vi "multi-mode-acquisition.vi"() -> ()   [LabVIEW 2014]
uses:
  camera test/SubVIs/Initilize Globals.vi
  <vilib>/vision/Image Controls.llb/IMAQ Image.ctl
  Glimpse-master/Glimpse core/Seq file v 1/Offset.ctl
  Glimpse-master/Glimpse core/Seq file v 1/file number.ctl
  Glimpse-master/Glimpse core/Seq file v 1/Offset table.ctl
  camera test/SubVIs/ctt's/Video acquisition state1.ctl
  Shutter Control/Shutter SubVis/Global Shutter Variables - SubVI.vi
  Shutter Control/Shutter SubVis/user event shutter global.ctl
  Shutter Control/Shutter SubVis/laser shutters.ctl
panel:
  in  "Max. number of acquisition files":i8(slide)=10 scale=0.0..50.0
  in  "Acquisition Protocol":T2(array[cluster])
  in  "Quit":bool
  in  "Start":bool
  in  "Acquisition Parameters":T3={"Readout Mode"=enum."Image", "Set Acquisition Mode"=enum."Single Scan", "Trigger Mode"=enum."Internal", "Exposure Time (s)"=1.0, "Accumulation Cycle (s)"=0.0, "Kinetic Cycle Time (s)"=1.0, "Number of Kinetics"=1, "Number of Accumulations"=1, "Set VS Speed"=1, "Pixel Rate"=enum."Standard CCD 3 Mhz 14 bits", "V Shift Amplitude"=enum."+1", "Preamp Gain"=enum."1.0"}
  in  "Image Size":T4={"H Bin"=1.0, "V Bin"=1.0, "Left"=1.0, "Right"=1024.0, "Top"=1.0, "Bottom"=1024.0} {"V Bin" min=0.0; "H Bin" min=0.0 step=1.0}
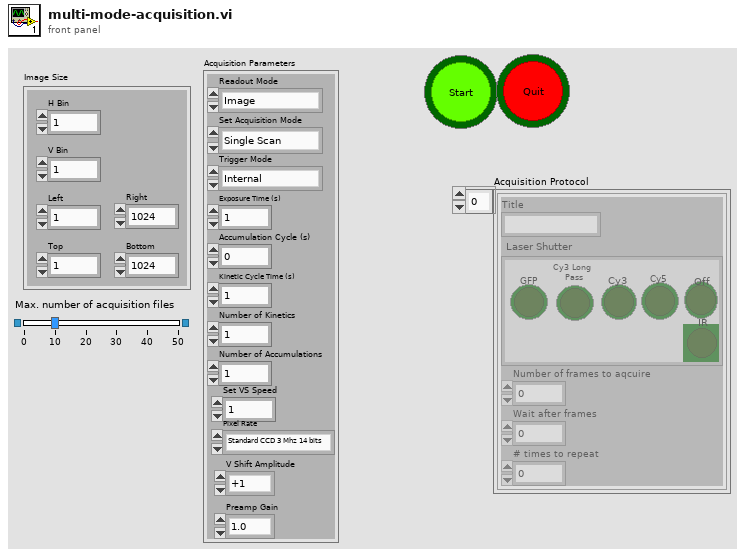
[diagram p1: front panel]
types:
  T1 = typedef "laser shutters.ctl" = enum32{"No Selection", "GFP", "Cy3 Long \nPass", "Cy3", "Cy5", "Off", "IR"}
  T2 = cluster{"Title":string, "Laser Shutter":T1, "Number of frames to aqcuire":dbl, "Wait after frames":dbl, "# times to repeat":dbl}[]
  T3 = cluster{"Readout Mode":enum16{"Full Vertical Binning", "Multi-Track", "Random-Track", "Single-Track", "Image"}, "Set Acquisition Mode":enum16{"(do nothing)", "Single Scan", "Accumulate", "Kinetics", "Fast Kinetics", "Run till abort"}, "Trigger Mode":enum16{"Internal", "External"}, "Exposure Time (s)":dbl, "Accumulation Cycle (s)":dbl, "Kinetic Cycle Time (s)":dbl, "Number of Kinetics":i32, "Number of Accumulations":i32, "Set VS Speed":i32, "Pixel Rate":enum16{"EM CCD 10 Mhz 14 bits", "EM CCD 5 Mhz 14 bits", "EM CCD 3 Mhz 14 bits", "EM CCD 1 Mhz 16 bits", "Standard CCD 3 Mhz 14 bits", "Standard CCD 1 Mhz 16 bits"}, "V Shift Amplitude":enum16{"normal", "+1", "+2", "+3", "+4"}, "Preamp Gain":enum16{"1.0", "2.4", "5.0"}}
  T4 = cluster{"H Bin":dbl, "V Bin":dbl, "Left":dbl, "Right":dbl, "Top":dbl, "Bottom":dbl}
  T5 = typedef "Video acquisition state1.ctl" = cluster{"Pixel depth":enum32{"8 bits", "16 bits", "Float", "Complex", "RGB Chunky", "Compressed"}, "Width":dbl, "Height":dbl, "Buffer":T6, "Frames Acquired":u32, "Time of 1st frame":dbl, "TTB element zero":u32, "File Offsets Array":T7, "TTB Array":u32[], "Sum Image (for averaging)":T6, "Time at end of last acquisition (ms)":u32, "Filter array":u16[], "Flow rate array":dbl[], "Temperature array":dbl[], "Field array":u16[], "Lasers array":u16[][], "Stage xyz array":dbl[][]}
  T6 = typedef "IMAQ Image.ctl" = refnum<image>
  T7 = typedef "Offset table.ctl" = cluster{"offset":T8, "file number":T9}[]
  T8 = typedef "Offset.ctl" = i32
  T9 = typedef "file number.ctl" = u8
  T10 = typedef "user event shutter global.ctl" = cluster{"Camera Shutter":bool, "Wheel Speed":u8, "Laser Shutter":enum32{"No Selection", "GFP", "Cy3 Long \nPass", "Cy3", "Cy5", "Off", "IR"}}
  T11 = cluster{"Frame Size (bytes)":i32, "Max Time (min)":i32, "Max Frames":i32, "Frames per acquisition file":i32, "Max time (s)":i32, "Max Space Req'd. (Gb)":dbl}
  T12 = typedef "acquisition control.ctl" = cluster{"H Bin":dbl, "V Bin":dbl, "Left":dbl, "Right":dbl, "Top":dbl, "Bottom":dbl}
  T13 = cluster{"Sequence files directory path":path, "Sequence files refnum array":refnum<file>[]}
  T14 = enum32{"No Selection", "GFP", "Cy3 Long \nPass", "Cy3", "Cy5", "Off", "IR"}
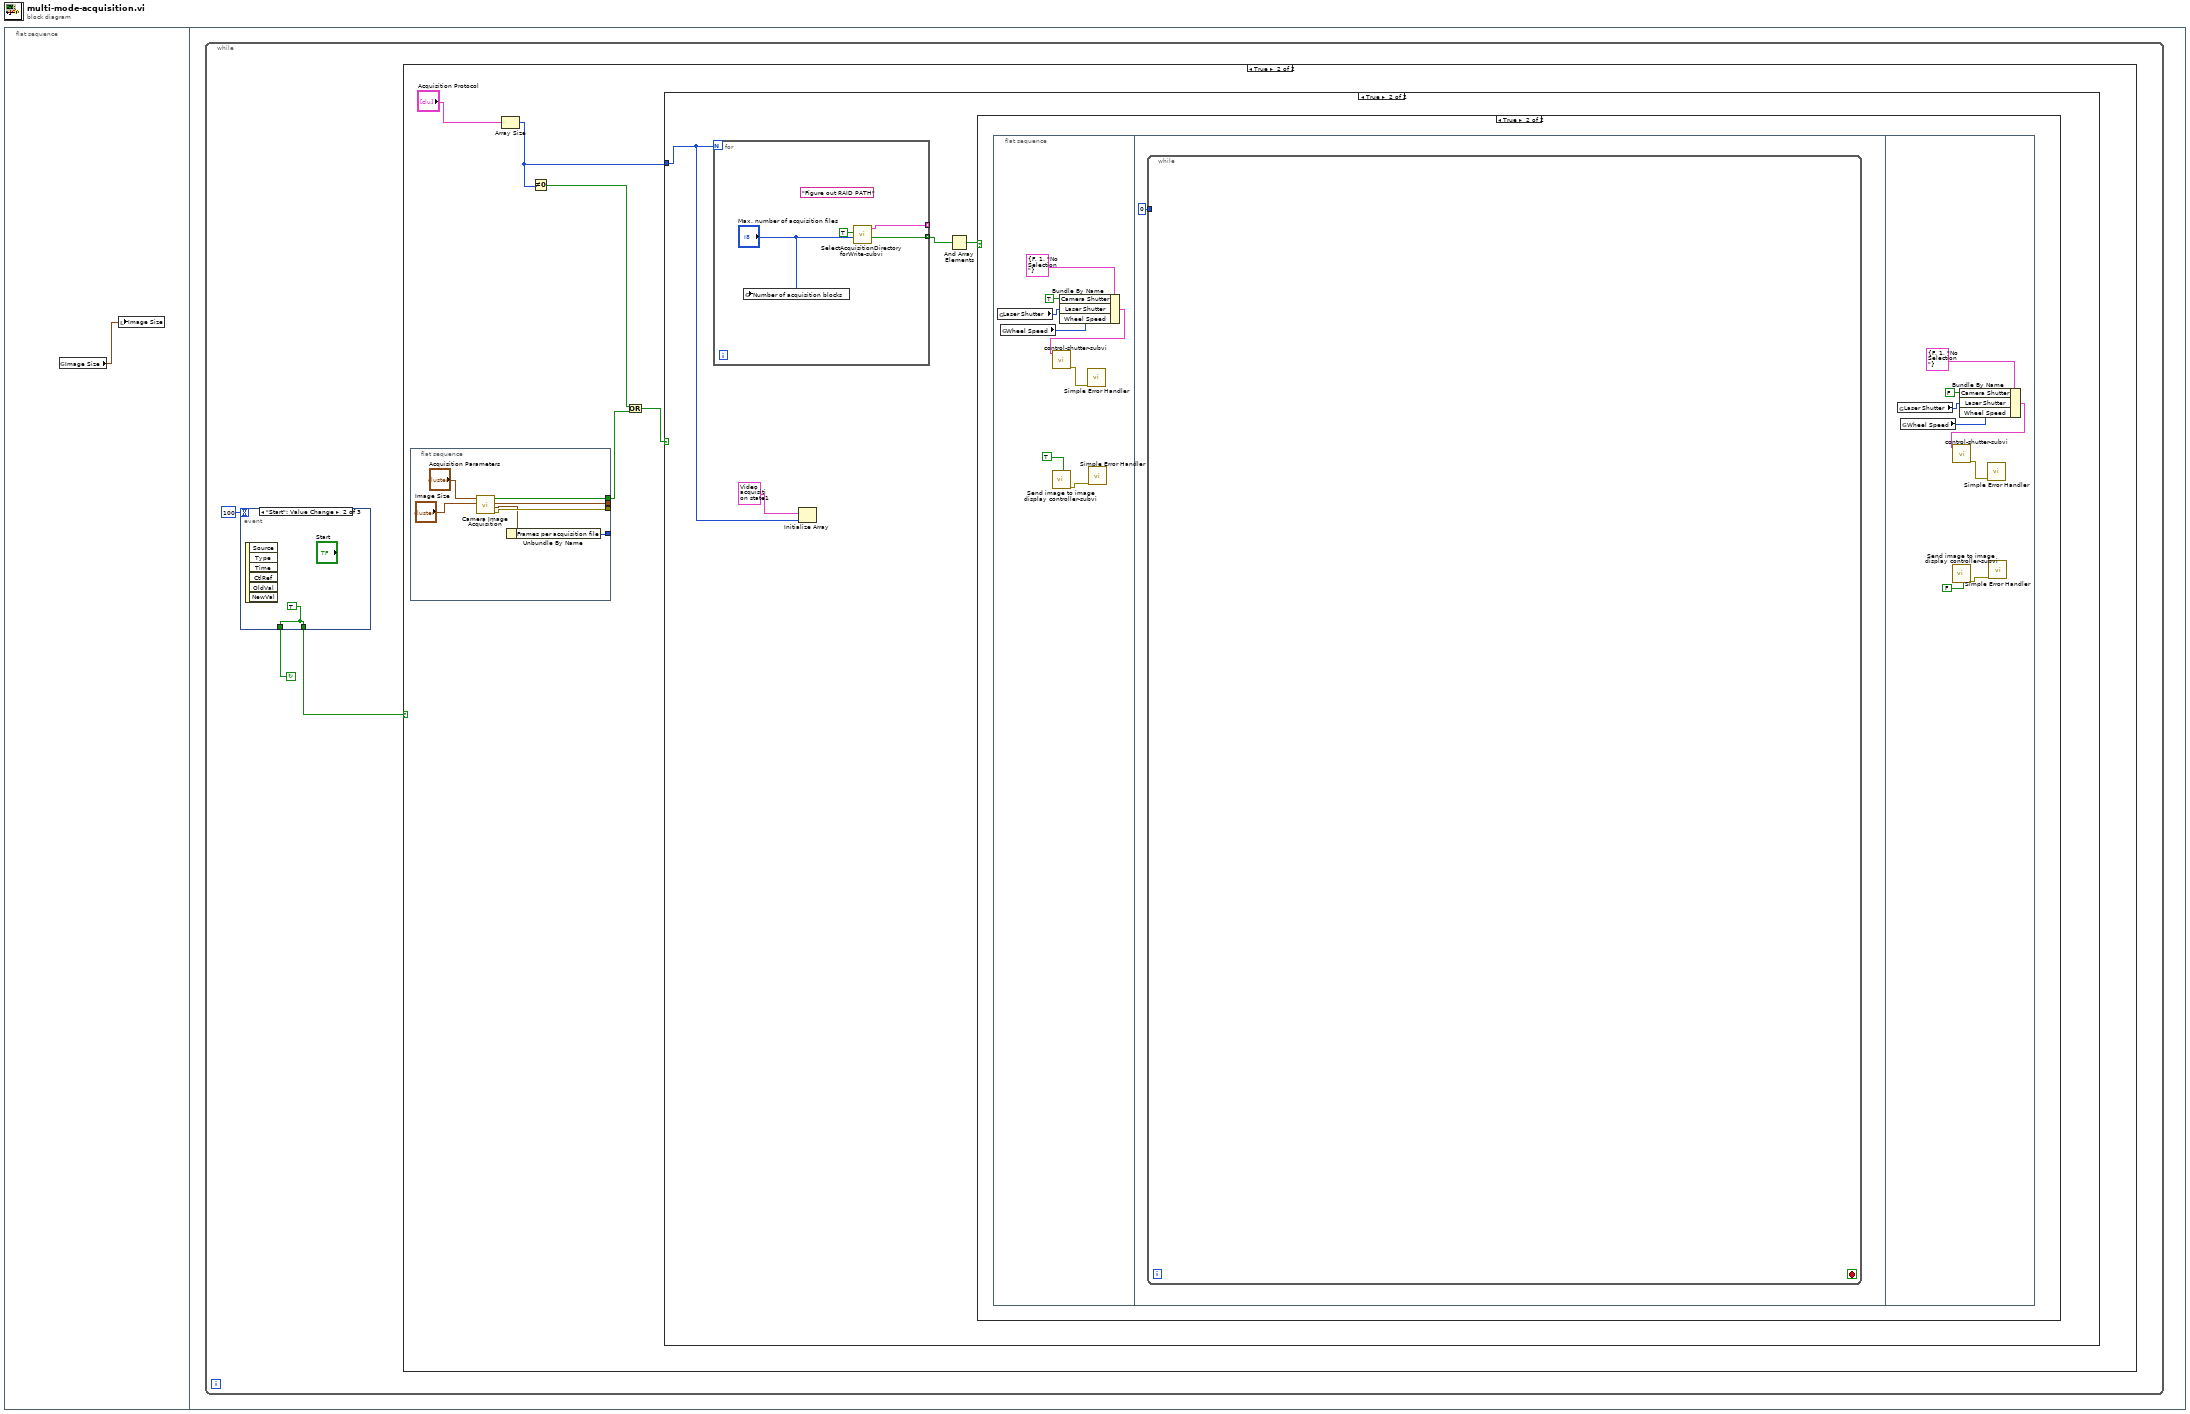
[diagram p0: block diagram]
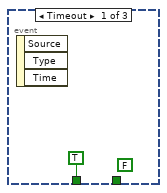
[diagram p5: hidden frame]
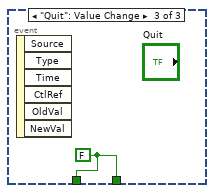
[diagram p6: hidden frame]
diagram:
  n1 = flat-sequence {
    frame #0 {
      n2 = global read "Initilize Globals.vi" "Image Size"() -> (w1:T4)
      n3 = local write "Image Size"(w1) -> ()
    }
    frame #1 {
      n4 = while {
        stop <- w3 continue-if-true
        n5 = event shown="[1] \"Start\": Value Change" {
          selector: _ -> [_ _ _]
          dyn-events: _ -> [_ _ _]
          timeout: 100 -> [_ _ _]
          tunnel: [TRUE w43 w44] -> w3
          tunnel: [_ w43 w44] -> w2
          event Timeout {
            (unwired) FALSE
            n6 = event-data() -> ()  [unwired: 1 in, 3 out]
          }
          event "Start": Value Change {
            w43 = TRUE
            n7 = event-data() -> ()  [unwired: 1 in, 6 out]
          }
          event "Quit": Value Change {
            w44 = FALSE
            n8 = event-data() -> ()  [unwired: 1 in, 6 out]
          }
        }
        n9 = case shown="True" w2 {
          frame False {
          }
          frame True {
            n10 = flat-sequence {
              tunnel: [w39] -> w7
              tunnel: [w38] -> _
              tunnel: [w36] -> _
              tunnel: [w35] -> _
              frame #0 {
                n11 = call "Camera Image Acquisition.vi"("Image Size"="Image Size", "Acquisition Parameters"="Acquisition Parameters") -> ("Error Out"=w38:errorcluster, "File properties"=w37:T11, "Image Size 2"=w36:T12, "Continue with acq?"=w39:bool)  [unwired: 6 in]
                n12 = Unbundle By Name(w37) -> ("Frames per acquisition file"=w35:i32)
              }
            }
            n13 = Array Size(array="Acquisition Protocol") -> (size(s)=w5:i32)
            n14 = Not Equal To 0?(x=w5) -> (x != 0?=w6:bool)
            n15 = Or(x=w6, y=w7) -> (x .or. y?=w8:bool)
            n16 = case shown="True" w8 {
              tunnel: w5 -> [_ w13]
              frame False {
              }
              frame True {
                n17 = for {
                  N: w13 -> [_]
                  tunnel: [w32] -> w11 mode=indexing
                  tunnel: [w31] -> _ mode=indexing
                  (unwired) "Figure out RAID PATH"
                  n18 = global write "Initilize Globals.vi" "Number of acquisition blocks"("Max. number of acquisition files") -> ()
                  n19 = call "SelectAcquisitionDirectoryforWrite-subvi.vi"("Number of acquisition files"="Max. number of acquisition files", "Autostart?"=TRUE) -> ("OK?"=w32:bool, "Sequence files handle"=w31:T13)  [unwired: 8 in]
                }
                n20 = Initialize Array(T5 {"Pixel depth"=enum."8 bits", "Width"=0.0, "Height"=0.0, "Buffer"=refnum, "Frames Acquired"=0, "Time of 1st frame"=0.0, "TTB element zero"=0, "File Offsets Array"=[], "TTB Array"=[], "Sum Image (for averaging)"=refnum, "Time at end of last acquisition (ms)"=0, "Filter array"=[], "Flow rate array"=[], "Temperature array"=[], "Field array"=[], "Lasers array"=[], "Stage xyz array"=[]} ("State"), w13) -> ()  [unwired: 1 out]
                n21 = And Array Elements(Boolean array=w11) -> (logical AND=w10:bool)
                n22 = case shown="True" w10 {
                  frame False {
                  }
                  frame True {
                    n23 = flat-sequence {
                      frame #0 {
                        n24 = global read "Global Shutter Variables - SubVI.vi" "Laser Shutter"() -> (w19:T14)
                        n25 = global read "Global Shutter Variables - SubVI.vi" "Wheel Speed"() -> (w18:u8)
                        n26 = call "Send image to image display controller-subvi.vi"("Start display controller?"=TRUE) -> ("error out"=w15:errorcluster)  [unwired: 8 in, 1 out]
                        n27 = Bundle By Name(cluster=T10 {"Camera Shutter"=FALSE, "Wheel Speed"=1, "Laser Shutter"=enum."No Selection"} ("Shutter Control"), "Camera Shutter"=TRUE, "Laser Shutter"=w19, "Wheel Speed"=w18) -> (w17:T10)
                        n28 = call "control-shutter-subvi.vi"("Shutter Control"=w17) -> ("Error Out"=w16:errorcluster)  [unwired: 10 in]
                        n29 = call <vilib>:"Simple Error Handler.vi"("error in (no error)"=w16) -> ()  [unwired: 1 in, 8 out]
                        n30 = call <vilib>:"Simple Error Handler.vi"("error in (no error)"=w15) -> ()  [unwired: 1 in, 8 out]
                      }
                      frame #1 {
                        n31 = while {
                          tunnel: 0 -> [_]
                          stop <- _ stop-if-true
                        }
                      }
                      frame #2 {
                        n32 = global read "Global Shutter Variables - SubVI.vi" "Laser Shutter"() -> (w28:T14)
                        n33 = global read "Global Shutter Variables - SubVI.vi" "Wheel Speed"() -> (w27:u8)
                        n34 = call "Send image to image display controller-subvi.vi"("Quit display controller?"=FALSE) -> ("error out"=w24:errorcluster)  [unwired: 8 in, 1 out]
                        n35 = Bundle By Name(cluster=T10 {"Camera Shutter"=FALSE, "Wheel Speed"=1, "Laser Shutter"=enum."No Selection"} ("Shutter Control"), "Camera Shutter"=FALSE, "Laser Shutter"=w28, "Wheel Speed"=w27) -> (w26:T10)
                        n36 = call "control-shutter-subvi.vi"("Shutter Control"=w26) -> ("Error Out"=w25:errorcluster)  [unwired: 10 in]
                        n37 = call <vilib>:"Simple Error Handler.vi"("error in (no error)"=w25) -> ()  [unwired: 1 in, 8 out]
                        n38 = call <vilib>:"Simple Error Handler.vi"("error in (no error)"=w24) -> ()  [unwired: 1 in, 8 out]
                      }
                    }
                  }
                }
              }
            }
          }
        }
      }
    }
  }
